vi "PrOM_TZCH_host.vi"() -> ()   [LabVIEW 2013]
uses:
  <instrlib>/niDCPower/nidcpower.llb/niDCPower Measurement Type.ctl
  <instrlib>/niDMM/nidmm.llb/niDMM Resolution in Digits.ctl
  <instrlib>/niDMM/nidmm.llb/niDMM Function.ctl
  <vilib>/Analysis/baseanly.llb/Mean (DBL).vi
  <instrlib>/niDMM/nidmm.llb/niDMM Configure Measurement Digits.vi
  <vilib>/Analysis/NI_AALBase.lvlib
panel:
  out "Счетчик сбоев":dbl
  in  "SEL sim":bool
  in  "Порог сбоя, мкА":dbl
  in  "Облучение!":bool=TRUE
  out "Photocurrent, uA":dbl
  out "refnum out":refnum<file>
  in  "Param_Log":path=path "D:/#rkm/Фонон-4/ТермоЛазер/Фонон-4_ПОМ_ПрОМ/Прога/ThermoLaser/Logs/Отчетные/ТЗЧ"
  out "Photodiode Current, uA":dbl(graph)=1.0181807397202647
  out "4071(2)_adress":refnum<k15>="PXI1Slot4_2 (12)" caption="4071(2)_out"
  in  "4071(2)":refnum<k15>="PXI1Slot4_2"
  in  "measurement type":T1=1 items=["Current", "Voltage"]
  out "measurement":dbl=4.999233750989324 format="%_6g"
  out "Enum":enum16{"Инициализация", "Ожидание", "Выход"}(ring)=enum."Выход"
  out "Выполняется":bool
  in  "stop":bool
  out "instrument handle out":refnum<k15>="PXI1Slot6 (9)"
  in  "Source_2-PD":refnum<k15>="PXI1Slot6" caption="Source_2"
  out "Ион":string="Хренон"
  out "Сеанс":i32=1
  out "Образец":i32=9
  out "Температура":i32=25
  # "НЕ ЗАБУДЬ УБРАТЬ ЖЕЛТЫЙ ДЖАМПЕР\nС А2"
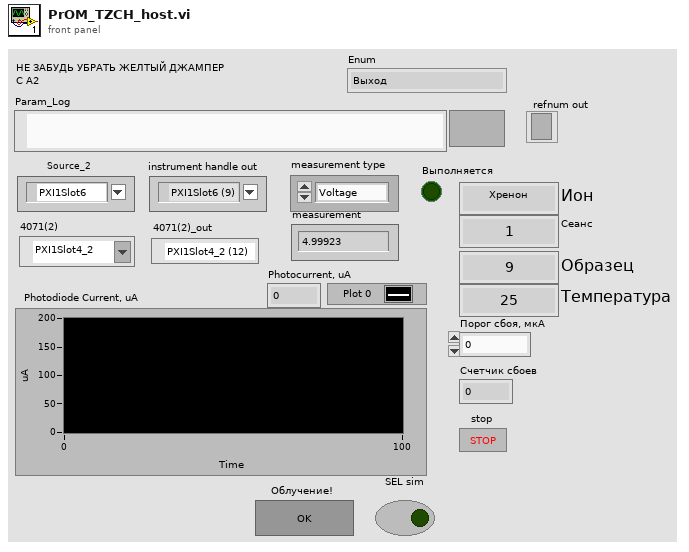
[diagram p1: front panel]
types:
  T1 = typedef "niDCPower Measurement Type.ctl" = i32
  T2 = typedef "niDMM Function.ctl" = enum16{"DC Volts", "AC Volts", "DC Current", "AC Current", "2-wire Resistance", "4-wire Resistance", "Diode", "Frequency", "Period", "AC Volts DC Coupled", "Capacitance", "Inductance", "Temperature"}
  T3 = enum16{"open", "replace", "create", "open or create", "replace or create", "replace or create with confirmation"}
  T4 = typedef "niDMM Resolution in Digits.ctl" = dbl
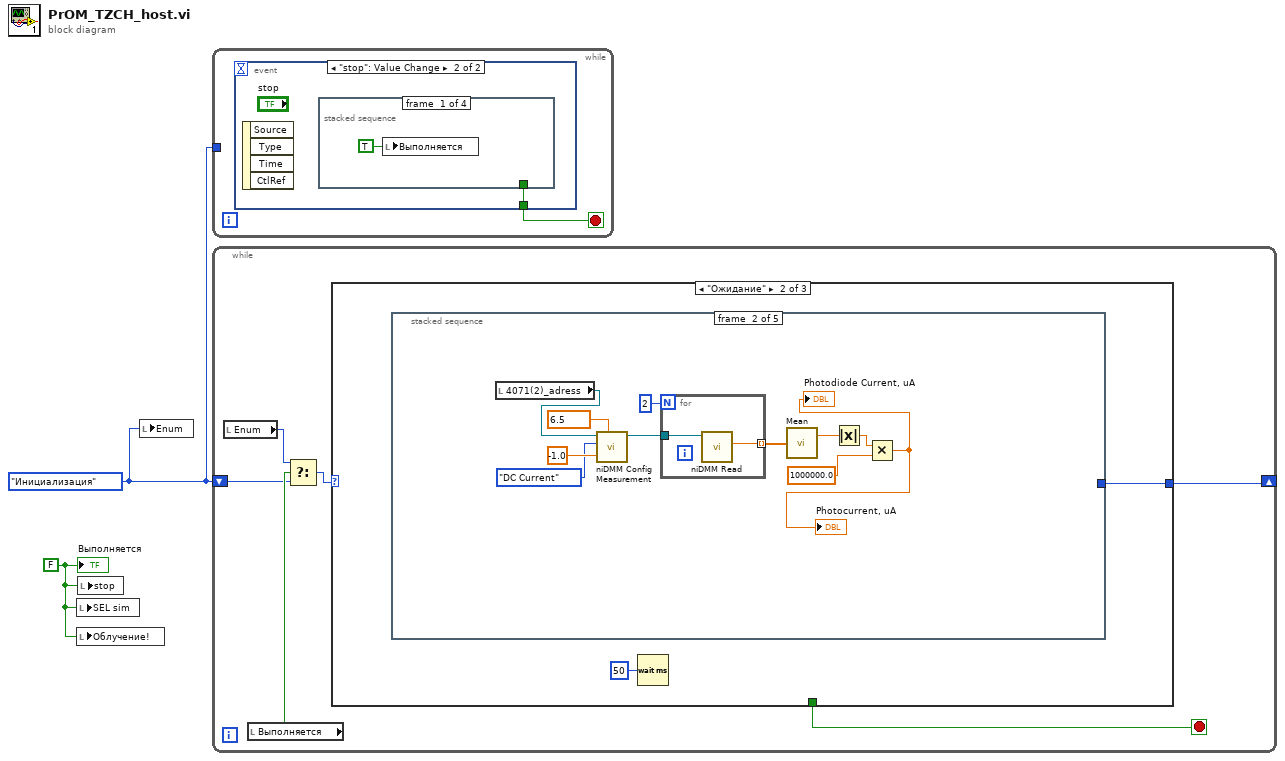
[diagram p0: block diagram]
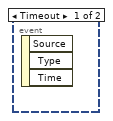
[diagram p2: hidden frame]
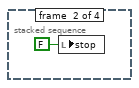
[diagram p3: hidden frame]
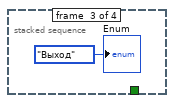
[diagram p4: hidden frame]
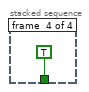
[diagram p5: hidden frame]
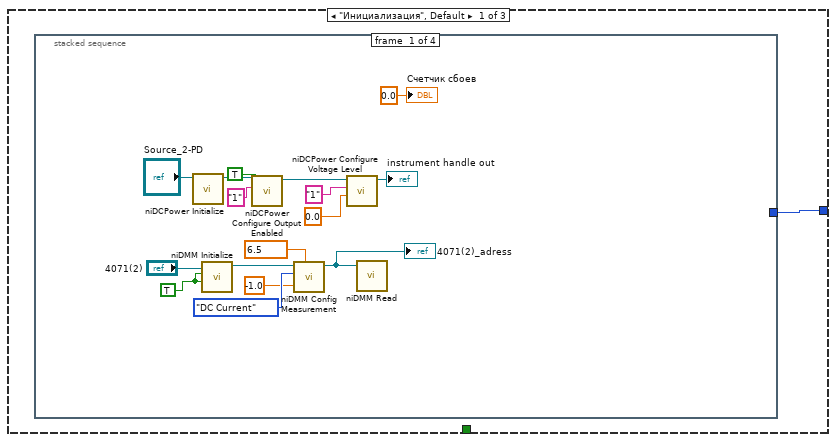
[diagram p6: hidden frame]
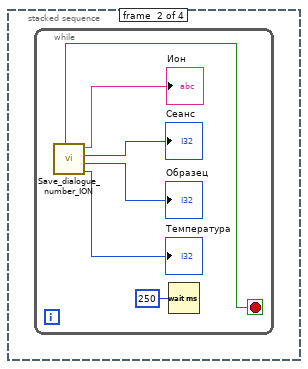
[diagram p7: hidden frame]
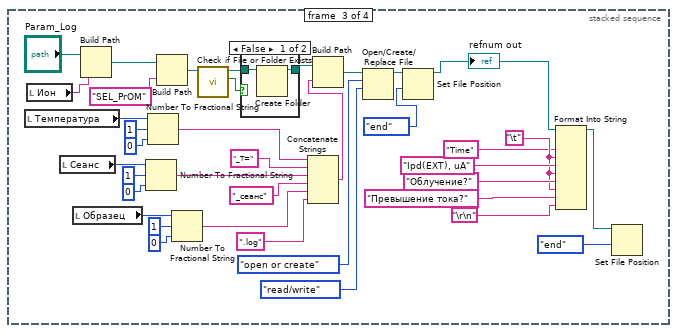
[diagram p8: hidden frame]
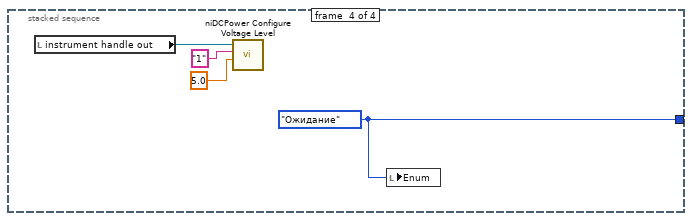
[diagram p10: hidden frame]
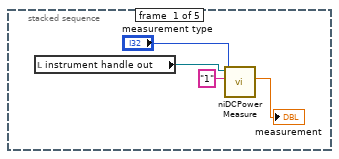
[diagram p11: hidden frame]
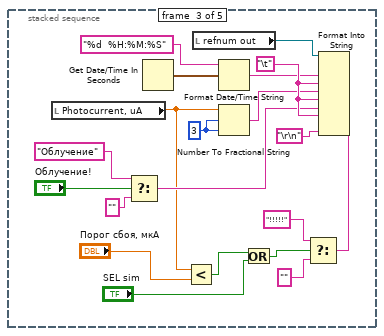
[diagram p12: hidden frame]
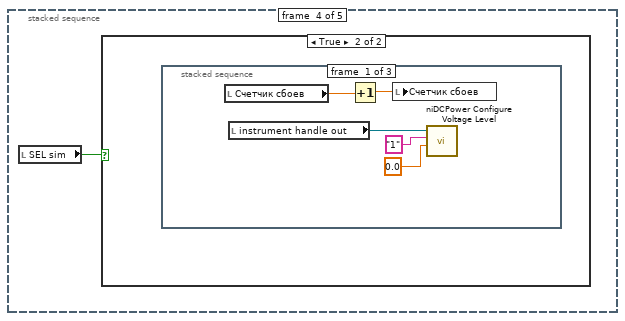
[diagram p13: hidden frame]
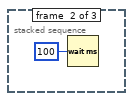
[diagram p15: hidden frame]
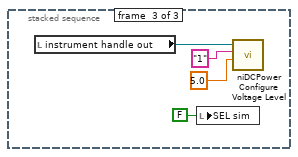
[diagram p16: hidden frame]
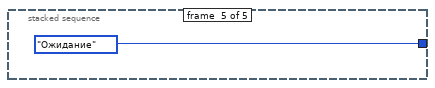
[diagram p17: hidden frame]
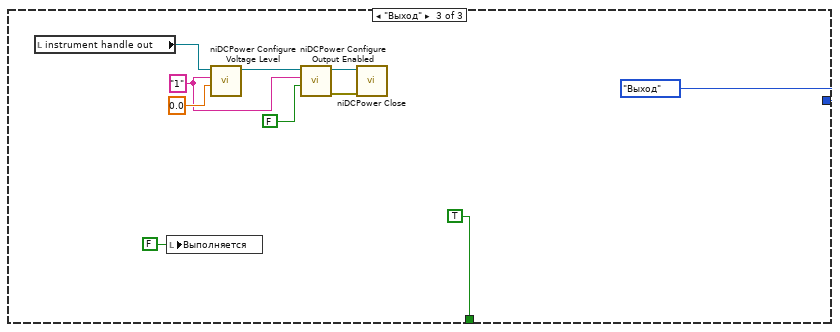
[diagram p18: hidden frame]
diagram:
  w1 = FALSE ("Выполняется")
  w2 = enum16{"Инициализация", "Ожидание", "Выход"}."Инициализация"
  n1 = local write "SEL sim"(w1) -> ()
  n2 = local write "Облучение!"(w1) -> ()
  n3 = local write "stop"(w1) -> ()
  n4 = local write "Enum"(w2) -> ()
  n5 = while {
    tunnel: w2 -> [_]
    stop <- w3 stop-if-true
    n6 = event shown="[1] \"stop\": Value Change" {
      selector: _ -> [_ _]
      dyn-events: _ -> [_ _]
      timeout: _ -> [_ _]
      tunnel: [_ w4] -> w3
      event Timeout {
        n7 = event-data() -> ()  [unwired: 1 in, 3 out]
      }
      event "stop": Value Change {
        n8 = event-data() -> ()  [unwired: 1 in, 4 out]
        n9 = stacked-sequence {
          tunnel: [_ _ _ TRUE] -> w4
          frame #0 {
            n10 = local write "Выполняется"(TRUE ("Выполняется")) -> ()
          }
          frame #1 {
            n11 = local write "stop"(FALSE ("stop")) -> ()
          }
          frame #2 {
            "Enum" <- enum16{"Инициализация", "Ожидание", "Выход"}."Выход" ("Enum")
          }
          frame #3 {
          }
        }
      }
    }
  }
  n12 = while {
    shift-right: [w14] -> _
    shift-left: w2 -> [w9]
    stop <- w11 stop-if-true
    n13 = local read "Enum"() -> (w10:enum16{"Инициализация", "Ожидание", "Выход"})
    n14 = local read "Выполняется"() -> (w13:bool)
    n15 = Select(t=w10, s=w13, f=w9) -> (s? t:f=w12:enum16{"Инициализация", "Ожидание", "Выход"})
    n16 = case shown="\"Ожидание\"" w12 {
      tunnel: [w15 w83 enum16{"Инициализация", "Ожидание", "Выход"}."Выход"] -> w14
      tunnel: [_ _ TRUE] -> w11
      frame "Инициализация", Default {
        n17 = stacked-sequence {
          tunnel: [_ _ _ w79] -> w15
          frame #0 {
            w17 = T4 6.5 items=["3 1/2"=3.5, "4 1/2"=4.5, "5 1/2"=5.5, "6 1/2"=6.5, "7 1/2"=7.5] ("Resolution in Digits")
            w22 = TRUE ("Reset")
            n18 = call <instrlib>:"niDCPower Initialize.vi"("resource name"="Source_2-PD") -> ("instrument handle out"=w27:refnum<k15>)  [unwired: 3 in, 7 out]
            n19 = call <instrlib>:"niDMM Initialize.vi"("Reset"=w22, "ID Query"=w22, "Instrument Descriptor"="4071(2)") -> ("instrument handle out"=w20:refnum<k15>)  [unwired: 7 in, 1 out]
            n20 = call <instrlib>:"niDCPower Configure Output Enabled.vi"("output enabled"=TRUE, "channel name"="1", "instrument handle"=w27) -> ("instrument handle out"=w26:refnum<k15>)  [unwired: 7 in, 1 out]
            n21 = call-poly <instrlib>:"niDMM Config Measurement.vi"("Range"=-1.0 ("Configuration:Measurement Options:Max Frequency"), "Resolution in Digits"=w17, "Function"=niDMM_Function."DC Current" ("multimeter mode"), "instrument handle"=w20) -> ("instrument handle out"=w18:refnum<k15>)  [unwired: 6 in, 1 out]
            "4071(2)_adress" <- w18
            n22 = call <instrlib>:"niDCPower Configure Voltage Level.vi"("voltage level"=0.0, "channel name"="1", "instrument handle"=w26) -> ("instrument handle out"=→"instrument handle out":refnum<k15>)  [unwired: 7 in, 1 out]
            n23 = call <instrlib>:"niDMM Read.vi"("instrument handle"=w18) -> ()  [unwired: 8 in, 3 out]
            "Счетчик сбоев" <- 0.0 ("Счетчик сбоев")
          }
          frame #1 {
            n24 = while {
              stop <- w32 stop-if-true
              n25 = call "Save_dialogue_number_ION.vi"() -> ("Температура 2"=→"Температура":i32, "Номер образца 2"=→"Образец":i32, "Номер сеанса 2"=→"Сеанс":i32, "Ион 2"=→"Ион":string, "OK Button 2"=w32:bool)  [unwired: 5 in]
              n26 = Wait (ms)(milliseconds to wait=u32 250) -> ()  [unwired: 1 out]
            }
          }
          frame #2 {
            w41 = "\t"
            n27 = local read "Температура"() -> (w69:i32)
            n28 = local read "Ион"() -> (w68:string)
            n29 = local read "Сеанс"() -> (w70:i32)
            n30 = local read "Образец"() -> (w71:i32)
            n31 = Build Path(base path="Param_Log", name or relative path=w68) -> (appended path=w64:path)
            n32 = Number To Fractional String(number=w70, width (-)=i16 1, precision (6)=i16 0) -> (F-format string=w57:string)  [unwired: 1 in]
            n33 = Number To Fractional String(number=w69, width (-)=i16 1, precision (6)=i16 0) -> (F-format string=w54:string)  [unwired: 1 in]
            n34 = Build Path(base path=w64, name or relative path="SEL_PrOM") -> (appended path=w62:path)
            n35 = Number To Fractional String(number=w71, width (-)=i16 1, precision (6)=i16 0) -> (F-format string=w60:string)  [unwired: 1 in]
            n36 = call <vilib>:"Check if File or Folder Exists.vi"("path"=w62) -> ("file or folder exists?"=w44:bool, "dup path"=w45:path)  [unwired: 8 in, 1 out]
            n37 = case shown="False" w44 {
              tunnel: w45 -> [w77 w78]
              tunnel: [w76 w78] -> w46
              frame False {
                n38 = Create Folder(path (use dialog)=w77) -> (created path=w76:path)  [unwired: 2 in, 2 out]
              }
              frame True {
              }
            }
            n39 = Concatenate Strings(w54, "_T=" ("string"), w57, "_сеанс" ("string"), w60, ".log" ("string")) -> (w65:string)
            n40 = Build Path(base path=w46, name or relative path=w65) -> (appended path=w47:path)
            n41 = Open/Create/Replace File(file path (use dialog)=w47, operation (0:open)=T3."open or create", access (0:read/write)=enum16{"read/write", "read-only", "write-only"}."read/write") -> (refnum out=w61:refnum<file>)  [unwired: 3 in, 2 out]
            n42 = Set File Position(refnum=w61, from (0:start)=enum16{"start", "end", "current"}."end") -> (refnum out=w67:refnum<file>)  [unwired: 2 in, 1 out]
            "refnum out" <- w67
            n43 = Format Into String(initial string=w67, "Time" ("input 1"), w41, "Ipd(EXT), uA", w41, "Облучение?", w41, "Превышение тока?", "\r\n") -> (resulting string=w40:refnum<file>)  [unwired: 2 in, 1 out]
            n44 = Set File Position(refnum=w40, from (0:start)=enum16{"start", "end", "current"}."end") -> ()  [unwired: 2 in, 2 out]
          }
          frame #3 {
            w79 = enum16{"Инициализация", "Ожидание", "Выход"}."Ожидание"
            n45 = local read "instrument handle out"() -> (w80:refnum<k15>)
            n46 = call <instrlib>:"niDCPower Configure Voltage Level.vi"("voltage level"=5.0, "channel name"="1", "instrument handle"=w80) -> ()  [unwired: 7 in, 2 out]
            n47 = local write "Enum"(w79) -> ()
          }
        }
      }
      frame "Ожидание" {
        n48 = stacked-sequence {
          tunnel: [_ _ _ _ enum16{"Инициализация", "Ожидание", "Выход"}."Ожидание"] -> w83
          frame #0 {
            n49 = local read "instrument handle out"() -> (w88:refnum<k15>)
            n50 = call <instrlib>:"niDCPower Measure.vi"("measurement type"="measurement type", "channel name"="1", "instrument handle"=w88) -> ("measurement"=→"measurement":dbl)  [unwired: 6 in, 2 out]
          }
          frame #1 {
            w97 = T4 6.5 items=["3 1/2"=3.5, "4 1/2"=4.5, "5 1/2"=5.5, "6 1/2"=6.5, "7 1/2"=7.5] ("Resolution in Digits")
            n51 = local read "4071(2)_adress"() -> (w90:refnum<k15>)
            n52 = call-poly <instrlib>:"niDMM Config Measurement.vi"("Range"=-1.0 ("Configuration:Measurement Options:Max Frequency"), "Resolution in Digits"=w97, "Function"=niDMM_Function."DC Current" ("multimeter mode"), "instrument handle"=w90) -> ("instrument handle out"=w96:refnum<k15>)  [unwired: 6 in, 1 out]
            n53 = for {
              N: 2 -> [_]
              tunnel: w96 -> [w101]
              tunnel: [w100] -> w94 mode=indexing
              n54 = call <instrlib>:"niDMM Read.vi"("instrument handle"=w101) -> ("Measurement"=w100:dbl)  [unwired: 8 in, 2 out]
            }
            n55 = call-poly <vilib>:"Mean.vi"("X"=w94) -> ("mean"=w93:dbl)  [unwired: 1 out]
            n56 = Absolute Value(x=w93) -> (abs(x)=w92:dbl)
            n57 = Multiply(x=w92, y=1000000.0) -> (x*y=→"Photodiode Current, uA" →"Photocurrent, uA":dbl)
          }
          frame #2 {
            w121 = "\t"
            w113 = i16 3 ("width (-)")
            n58 = local read "Photocurrent, uA"() -> (w106:dbl)
            n59 = Select(t="Облучение", s="Облучение!", f="") -> (s? t:f=w112:string)
            n60 = Get Date/Time In Seconds() -> (seconds since 1Jan1904=w115:timestamp)
            n61 = Less?(x=w106, y="Порог сбоя, мкА") -> (x < y?=w102:bool)
            n62 = local read "refnum out"() -> (w107:refnum<file>)
            n63 = Format Date/Time String(time format string (%c)="%d  %H:%M:%S", seconds (now)=w115) -> (date/time string=w116:string)  [unwired: 1 in]
            n64 = Number To Fractional String(number=w106, width (-)=w113, precision (6)=w113) -> (F-format string=w117:string)  [unwired: 1 in]
            n65 = Or(x=w102, y="SEL sim") -> (x .or. y?=w104:bool)
            n66 = Select(t="!!!!!", s=w104, f="") -> (s? t:f=w109:string)
            n67 = Format Into String(initial string=w107, w116, w121, w117, w121, w112, w121, w109, "\r\n") -> ()  [unwired: 2 in, 2 out]
          }
          frame #3 {
            n68 = local read "SEL sim"() -> (w122:bool)
            n69 = case shown="True" w122 {
              frame False {
              }
              frame True {
                n70 = stacked-sequence {
                  frame #0 {
                    n71 = local read "Счетчик сбоев"() -> (w126:dbl)
                    n72 = local read "instrument handle out"() -> (w123:refnum<k15>)
                    n73 = Increment(x=w126) -> (x+1=w127:dbl)
                    n74 = local write "Счетчик сбоев"(w127) -> ()
                    n75 = call <instrlib>:"niDCPower Configure Voltage Level.vi"("voltage level"=0.0, "channel name"="1", "instrument handle"=w123) -> ()  [unwired: 7 in, 2 out]
                  }
                  frame #1 {
                    n76 = Wait (ms)(milliseconds to wait=u32 100) -> ()  [unwired: 1 out]
                  }
                  frame #2 {
                    n77 = local read "instrument handle out"() -> (w130:refnum<k15>)
                    n78 = local write "SEL sim"(FALSE) -> ()
                    n79 = call <instrlib>:"niDCPower Configure Voltage Level.vi"("voltage level"=5.0, "channel name"="1", "instrument handle"=w130) -> ()  [unwired: 7 in, 2 out]
                  }
                }
              }
            }
          }
          frame #4 {
          }
        }
        n80 = Wait (ms)(milliseconds to wait=u32 50) -> ()  [unwired: 1 out]
      }
      frame "Выход" {
        w134 = "1" ("channel name")
        n81 = local read "instrument handle out"() -> (w137:refnum<k15>)
        n82 = local write "Выполняется"(FALSE ("Выполняется")) -> ()
        n83 = call <instrlib>:"niDCPower Configure Voltage Level.vi"("voltage level"=0.0, "channel name"=w134, "instrument handle"=w137) -> ("instrument handle out"=w138:refnum<k15>)  [unwired: 7 in, 1 out]
        n84 = call <instrlib>:"niDCPower Configure Output Enabled.vi"("output enabled"=FALSE, "channel name"=w134, "instrument handle"=w138) -> ("error out"=w136:errorcluster, "instrument handle out"=w135:refnum<k15>)  [unwired: 7 in]
        n85 = call <instrlib>:"niDCPower Close.vi"("error in (no error)"=w136, "instrument handle"=w135) -> ()  [unwired: 9 in, 1 out]
      }
    }
  }
  "Выполняется" <- w1
